vi "Load Plot Data.vi"(11 "Graph":refnum<vi>[](array[refnum])) -> ()   [LabVIEW 2020]
uses:
  <vilib>/Utility/NIReport.llb/Report Type.ctl
  <vilib>/addons/_office/excel.llb/Excel Get Data ([str]).vi
  <vilib>/Utility/NIReport.llb/NI_report.lvclass
  <vilib>/Utility/NIReport.llb/NI_ReportGenerationCore.lvlib
  <vilib>/addons/_office/NI_ReportGenerationToolkit.lvlib
  <vilib>/Utility/NIReport.llb/Excel/NI_Excel.lvclass
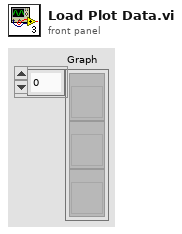
[diagram p1: front panel]
types:
  T1 = typedef "NI_ReportGenerationCore.lvlib/Report Type.ctl" = enum16{"HTML", "Word", "Excel"}
  T2 = enum16{"maximized", "minimized", "normal", "no change"}
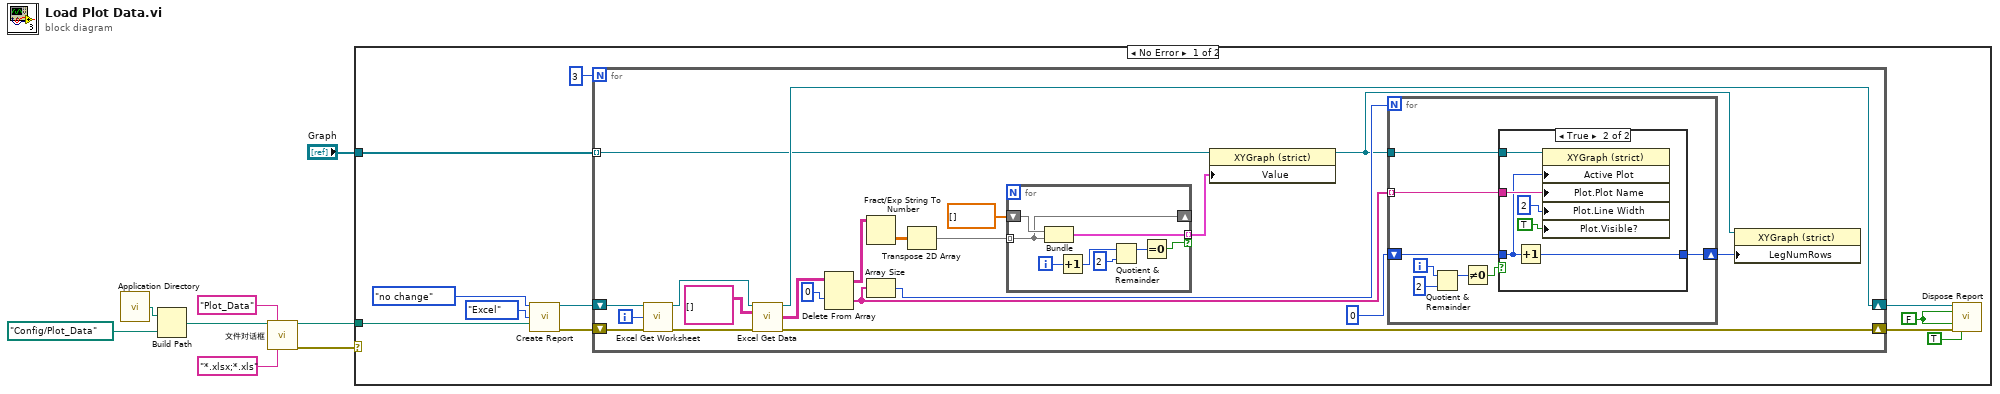
[diagram p0: block diagram]
diagram:
  n1 = call <vilib>:"Application Directory.vi"() -> ("Application Directory"=w7:path)
  n2 = Build Path(base path=w7, name or relative path=path "Config/Plot_Data") -> (appended path=w8:path)
  n3 = call "文件对话框"("start path"=w8, "prompt"="Plot_Data" ("default name"), "pattern (all files)"="*.xlsx;*.xls") -> ("selected path"=w2:path, "error out"=w3:errorcluster)  [unwired: 9 in, 2 out]
  n4 = case shown="No Error" w3 {
    tunnel: w2 -> [w18 _]
    tunnel: "Graph" -> [w9 _]
    frame No Error {
      w11 = FALSE ("wait until printing completed? (T)")
      n5 = call <vilib>:"Create Report.vi"("window state (normal)"=T2."no change", "report type"=Report_Type."Excel", "template (empty)"=w18) -> ("report out"=w16:refnum<class "NI_report.lvclass">, "error out"=w15:errorcluster)  [unwired: 11 in]
      n6 = for {
        N: 3 -> [_]
        shift-right: [w35] -> w13
        shift-left: w16 -> [w38]
        shift-right: [w36] -> w14
        shift-left: w15 -> [w37]
        tunnel: w9 -> [w20] mode=indexing
        i -> [w34]
        n7 = call <vilib>:"Excel Get Worksheet.vi"("report in"=w38, "worksheet index (0)"=w34, "error in (no error)"=w37) -> ("report out"=w40:refnum<class "NI_report.lvclass">, "error out"=w39:errorcluster)  [unwired: 11 in]
        n8 = call-poly <vilib>:"Excel Get Data.vi"("report in"=w40, "data type"=string[][] [], "error in (no error)"=w39) -> ("report out"=w35:refnum<class "NI_report.lvclass">, "data"=w30:string[][], "error out"=w36:errorcluster)  [unwired: 10 in]
        n9 = Delete From Array(array=w30, index (row)=0) -> (deleted portion=w22:string[], array with subset deleted=w31:string[][])  [unwired: 2 in]
        n10 = Fract/Exp String To Number(string=w31) -> (number=w29:dbl[][])  [unwired: 3 in, 1 out]
        n11 = Array Size(array=w22) -> (size(s)=w25:i32)
        n12 = Transpose 2D Array(2D array=w29) -> (transposed array=w27:dbl[][])
        n13 = for {
          tunnel: w27 -> [w62] mode=indexing
          shift-right: [w62] -> _
          shift-left: dbl[] [] -> [w63]
          tunnel: [w61] -> w26 mode=indexing if=w56
          i -> [w60]
          n14 = Bundle(w63, w62) -> (w61:cluster{dbl[], dbl[]})  [unwired: 1 in]
          n15 = Increment(x=w60) -> (x+1=w58:i32)
          n16 = Quotient & Remainder(x=w58, y=2 ("x")) -> (x-y*floor(x/y)=w57:i32)  [unwired: 1 out]
          n17 = Equal To 0?(x=w57) -> (x = 0?=w56:bool)
        }
        n18 = property class="XYGraph (strict)"(reference=w20, "Value"=w26) -> (reference out=w21:refnum<vi>)  [unwired: 1 in, 1 out]
        n19 = for {
          N: w25 -> [_]
          tunnel: w22 -> [w44] mode=indexing
          shift-right: [w42] -> w24
          shift-left: 0 ("x") -> [w43]
          tunnel: w21 -> [w41]
          i -> [w47]
          n20 = Quotient & Remainder(x=w47, y=2 ("x")) -> (x-y*floor(x/y)=w46:i32)  [unwired: 1 out]
          n21 = Not Equal To 0?(x=w46) -> (x != 0?=w45:bool)
          n22 = case shown="True" w45 {
            tunnel: w44 -> [_ w54]
            tunnel: w43 -> [w49 w53]
            tunnel: [w49 w52] -> w42
            tunnel: w41 -> [_ w50]
            frame False {
            }
            frame True {
              n23 = Increment(x=w53) -> (x+1=w52:i32)
              n24 = property on="Property Node" class="XYGraph (strict)"(reference=w50, "Active Plot"=w53, "Plot.Plot Name"=w54, "Plot.Line Width"=u8 2, "Plot.Visible?"=TRUE ("Plot.Visible")) -> ()  [unwired: 1 in, 2 out]
            }
          }
        }
        n25 = property on="Property Node" class="XYGraph (strict)"(reference=w21, "LegNumRows"=w24) -> ()  [unwired: 1 in, 2 out]
      }
      n26 = call-dynamic "Dispose Report.vi"("report in"=w13, "wait until printing completed? (T)"=w11, "save changes? (F)"=w11, "error in (no error)"=w14, "close report? (T)"=TRUE ("wait until printing completed? (T)")) -> ()  [unwired: 10 in, 1 out]
    }
    frame Error {
    }
  }
